vi "Main Abstraction Level 5.vi"() -> ()   [LabVIEW 2019]
doc: "This is one of the levels of abstract design along the timeline leading to the goal of a complete measurement application."
uses:
  messages/MeasureAndLogMessage.lvclass/MeasureAndLogMessage.ctl
  subVIs/Measure and Log Settings.ctl
  subVIs/Simulated Signal Type.ctl
  <extravilib>/ChannelInstances/Stream-str/Read With Abort.vi
  <extravilib>/ChannelInstances/Lossy Stream-a[.](wfm(dbl))/Read With Abort.vi
  <resource>/Channels/Messenger/Read With Abort.vi
  <vilib>/ChannelSupport/Channel Message/Read ID.vi
  <extravilib>/ChannelInstances/Stream-a[.](wfm(dbl))/Read With Abort.vi
  <extravilib>/ChannelInstances/Stream-a[.](wfm(dbl))/Endpoint.vi
  <extravilib>/ChannelInstances/Stream-str/EndpointRead.vi
  <extravilib>/ChannelInstances/Lossy Stream-a[.](wfm(dbl))/EndpointRead.vi
  <extravilib>/ChannelInstances/Stream-a[.](wfm(dbl))/EndpointRead.vi
  <extravilib>/ChannelInstances/Lossy Stream-a[.](wfm(dbl))/Endpoint.vi
  <extravilib>/ChannelInstances/Stream-str/Endpoint.vi
  messages/MeasureAndLogMessage.lvclass
  e:/builds/penguin/labview/branches/2019/dev/dist/vi.lib/ChannelSupport/Channel Message/Channel Message.lvclass
  <extravilib>/ChannelInstances/Tag-path/Instantiate.vi
  <extravilib>/ChannelInstances/Stream-a[.](wfm(dbl))/Instantiate.vi
  <extravilib>/ChannelInstances/Lossy Stream-a[.](wfm(dbl))/Instantiate.vi
  <extravilib>/ChannelInstances/Lossy Stream-a[.](wfm(dbl))/)Channel.vi
  <resource>/ChannelSupport/_ChannelSupport/WaitIfNeeded.vi
  <extravilib>/ChannelInstances/Stream-str/Instantiate.vi
  <extravilib>/ChannelInstances/Stream-str/)Channel.vi
  <extravilib>/ChannelInstances/Tag-bool/Instantiate.vi
  <extravilib>/ChannelInstances/Tag-t'Measure and Log Settings.ctl'/Instantiate.vi
  <resource>/Channels/Messenger/Instantiate.vi
  <resource>/Channels/Messenger/Endpoint.vi
  <extravilib>/ChannelInstances/Tag-t'Measure and Log Settings.ctl'/Endpoint.vi
  <extravilib>/ChannelInstances/Tag-path/Endpoint.vi
  <extravilib>/ChannelInstances/Tag-bool/Endpoint.vi
  <extravilib>/ChannelInstances/Stream-a[.](wfm(dbl))/)Channel.vi
  <resource>/Channels/Messenger/Messenger.lvlib
  <extravilib>/ChannelInstances/Stream-str.lvlib
  <extravilib>/ChannelInstances/Lossy Stream-a[.](wfm(dbl)).lvlib
  <extravilib>/ChannelInstances/Tag-bool.lvlib
  <extravilib>/ChannelInstances/Stream-a[.](wfm(dbl)).lvlib
  <extravilib>/ChannelInstances/Tag-path.lvlib
  <extravilib>/ChannelInstances/Tag-t'Measure and Log Settings.ctl'.lvlib
panel:
  in  "Exit flag":bool
  in  "Record":bool
  in  "Stop":bool
  out "Data":waveform(dbl)[](graph)
  out "Status":string
  in  "Settings":bool
  in  "Start":bool
  in  "Exit":bool
  # "Continuous Measurement Data Logger"
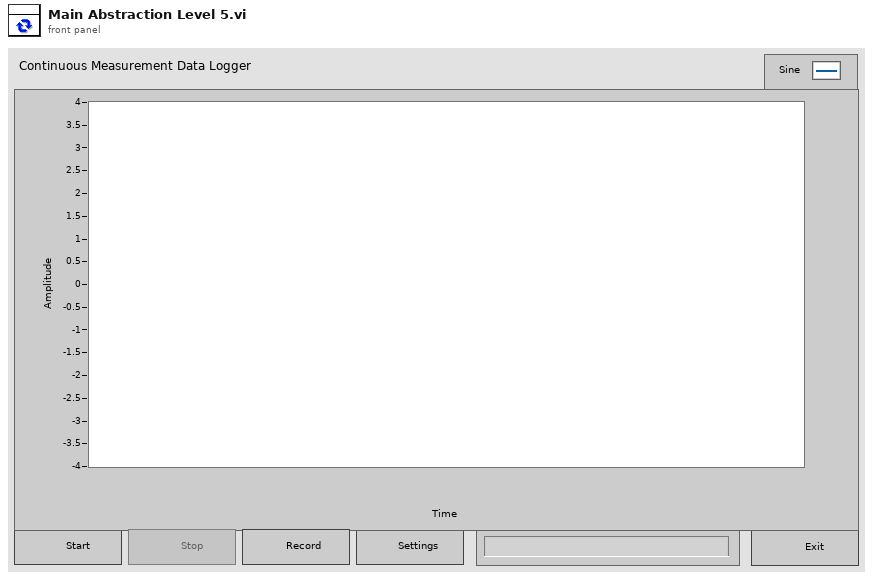
[diagram p1: front panel]
types:
  T1 = typedef "Measure and Log Settings.ctl" = cluster{"sample rate":dbl, "input range":dbl, "logfile path":path, "Simulated Signal":cluster{"signal type":T2, "frequency":dbl, "amplitude":dbl}}
  T2 = typedef "Simulated Signal Type.ctl" = enum16{"Sine Wave", "Square Wave with Noise"}
  T3 = enum8{"Enabled", "Disabled", "Disabled and Grayed Out"}
  T4 = typedef "Messenger.lvlib/))Channel.ctl" = refnum<queue>
  T5 = typedef "Tag-t'Measure and Log Settings.ctl'.lvlib/))Channel.ctl" = refnum<queue>
  T6 = typedef "Tag-path.lvlib/))Channel.ctl" = refnum<queue>
  T7 = typedef "Tag-bool.lvlib/))Channel.ctl" = refnum<queue>
  T8 = typedef "Stream-a[.](wfm(dbl)).lvlib/)Channel.ctl" = refnum<queue>
  T9 = typedef "Stream-str.lvlib/)Channel.ctl" = refnum<queue>
  T10 = typedef "Lossy Stream-a[.](wfm(dbl)).lvlib/)Channel.ctl" = refnum<queue>
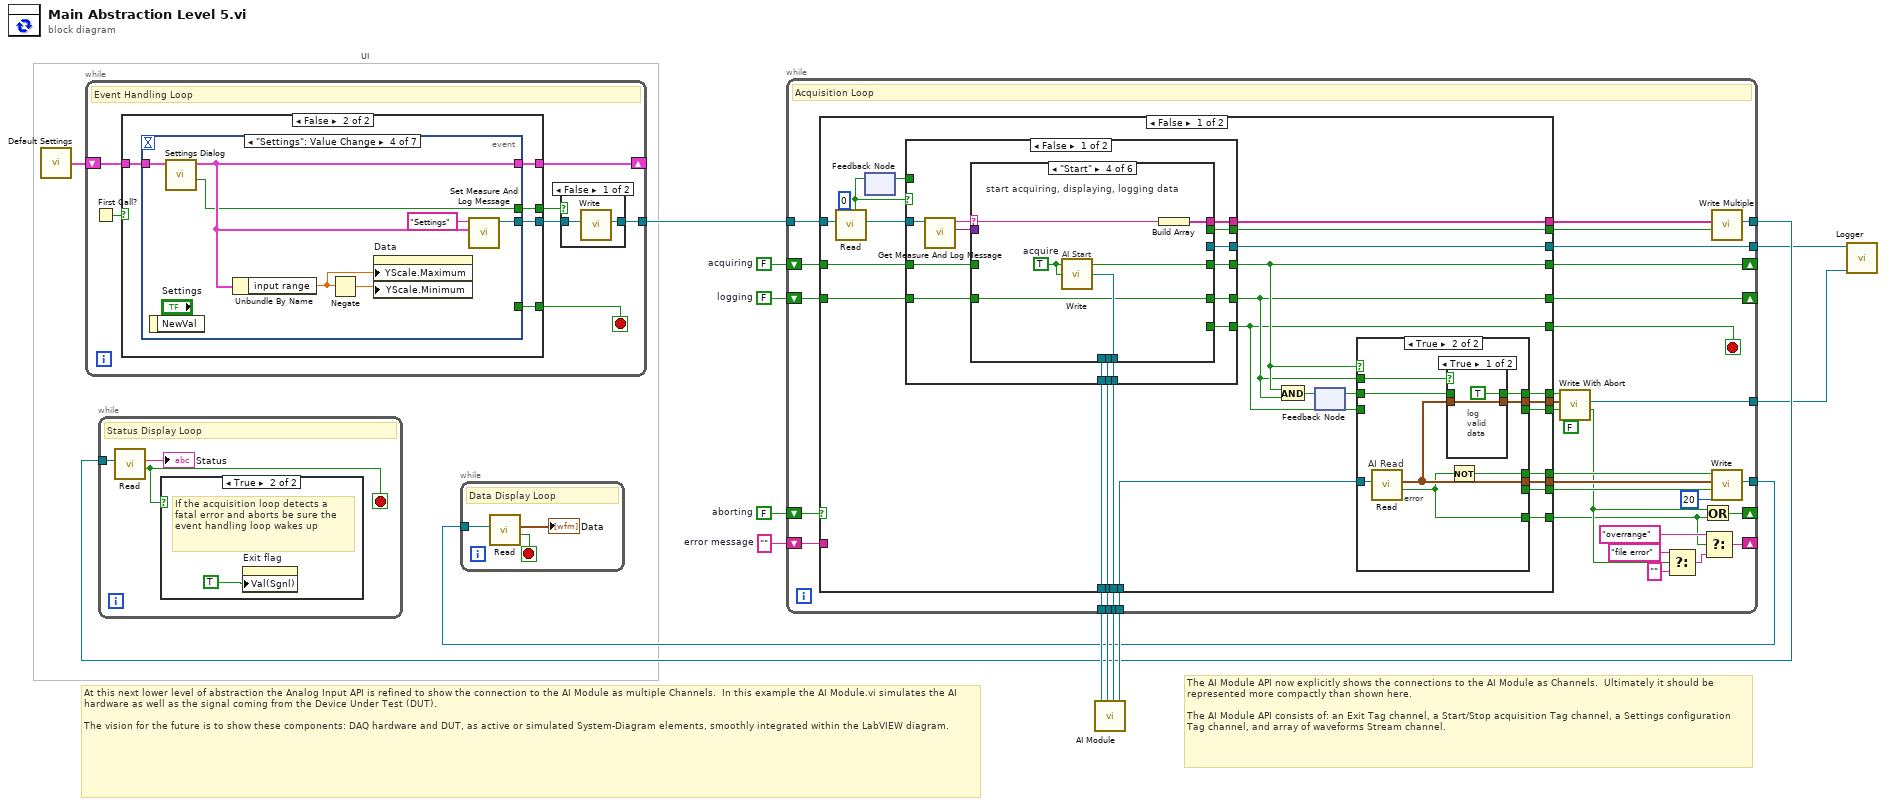
[diagram p0: block diagram]
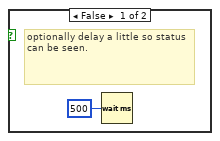
[diagram p2: hidden frame]
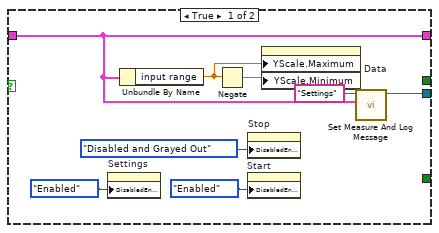
[diagram p3: hidden frame]
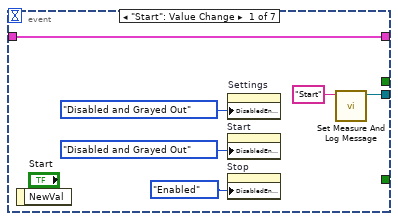
[diagram p4: hidden frame]
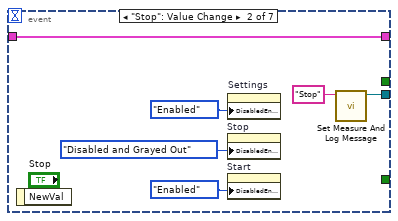
[diagram p5: hidden frame]
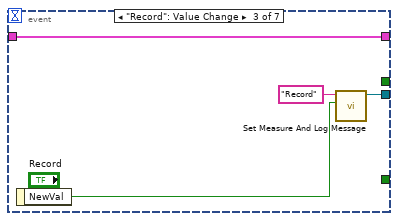
[diagram p6: hidden frame]
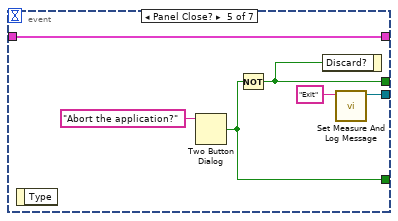
[diagram p7: hidden frame]
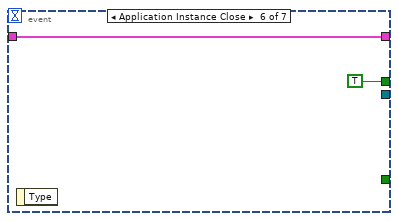
[diagram p8: hidden frame]
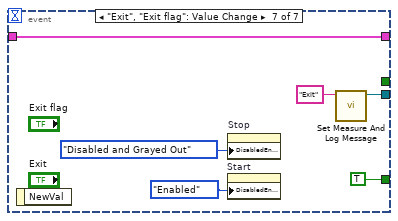
[diagram p9: hidden frame]
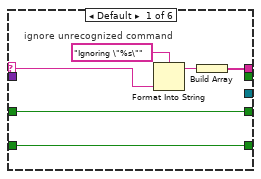
[diagram p11: hidden frame]
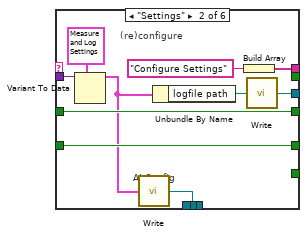
[diagram p12: hidden frame]
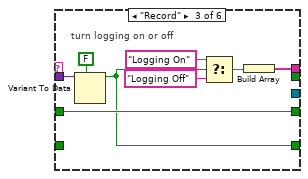
[diagram p13: hidden frame]
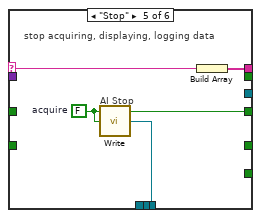
[diagram p14: hidden frame]
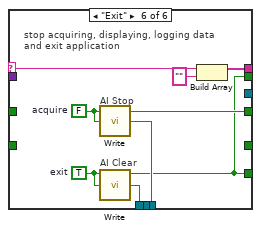
[diagram p15: hidden frame]
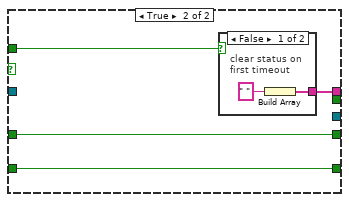
[diagram p16: hidden frame]
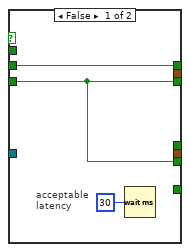
[diagram p18: hidden frame]
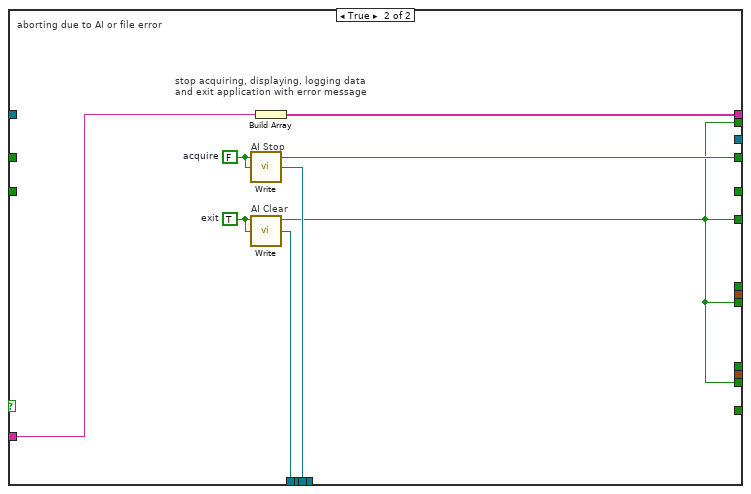
[diagram p20: hidden frame]
diagram:
  w8 = ""  # error message
  w10 = FALSE  # aborting
  w11 = FALSE  # logging
  w12 = FALSE  # acquiring
  # "At this next lower level of abstraction the Analog Input API is refined to show the connection to the AI Module as multiple Channels.  In this example the AI Module.vi simulates the AI hardware as well as the signal coming from the Device Under Test (DUT).\n\nThe vision for the future is to show these components: DAQ hardware and DUT, as active or simulated System-Diagram elements, smoothly integrated within the LabVIEW diagram."
  # "The AI Module API now explicitly shows the connections to the AI Module as Channels.  Ultimately it should be represented more compactly than shown here.\n\nThe AI Module API consists of: an Exit Tag channel, a Start/Stop acquisition Tag channel, a Settings configuration Tag channel, and array of waveforms Stream channel."
  # "UI"
  n1 = call "Default Settings.vi"() -> ("default settings"=w9:T1)
  n2 = while {
    tunnel: [w17] -> w13
    shift-right: [w20] -> _
    shift-left: w9 -> [w19]
    stop <- w21 stop-if-true
    # "Event Handling Loop"
    n3 = First Call?() -> (First Call?: T/F=w18:bool)
    n4 = case shown="False" w18 {
      tunnel: [_ w34] -> w21
      tunnel: [w28 w33] -> w20
      tunnel: w19 -> [w28 w32]
      tunnel: [w24 w31] -> w16
      tunnel: [_ w30] -> w15
      frame True {
        n5 = property on="Settings" class="Bool"("DisabledEnum"=T3."Enabled" ("Disabled")) -> ()  [unwired: 2 in, 2 out]
        n6 = Unbundle By Name(w28) -> ("input range"=w22:dbl)
        n7 = Negate(x=w22) -> (-x=w23:dbl)
        n8 = property on="Stop" class="Bool"("DisabledEnum"=T3."Disabled and Grayed Out" ("Disabled")) -> ()  [unwired: 2 in, 2 out]
        n9 = property on="Start" class="Bool"("DisabledEnum"=T3."Enabled" ("Disabled")) -> ()  [unwired: 2 in, 2 out]
        n10 = property on="Data" class="WFChart (strict)"("YScale.Maximum"=w22, "YScale.Minimum"=w23) -> ()  [unwired: 2 in, 2 out]
        n11 = call "Set Measure And Log Message.vi"("args"=w28, "command"="Settings") -> ("MyMessage"=w24:refnum<class "MeasureAndLogMessage.lvclass">)  [unwired: 9 in]
      }
      frame False {
        n12 = event shown="[3] \"Settings\": Value Change" {
          selector: _ -> [_ _ _ _ _ _ _]
          dyn-events: _ -> [_ _ _ _ _ _ _]
          timeout: _ -> [_ _ _ _ _ _ _]
          tunnel: [_ _ _ _ w59 _ TRUE] -> w34
          tunnel: [w36 w42 w48 w56 w62 w65 w67] -> w33
          tunnel: w32 -> [w36 w42 w48 w57 w62 w65 w67]
          tunnel: [w35 w41 w47 w55 w60 _ w66] -> w31
          tunnel: [_ _ _ w53 w58 TRUE ("cancelled") _] -> w30
          event "Start": Value Change {
            n13 = event-data() -> ()  [unwired: 1 in, 1 out]
            n14 = property on="Settings" class="Bool"("DisabledEnum"=T3."Disabled and Grayed Out" ("Disabled")) -> ()  [unwired: 2 in, 2 out]
            n15 = property on="Start" class="Bool"("DisabledEnum"=T3."Disabled and Grayed Out" ("Disabled")) -> ()  [unwired: 2 in, 2 out]
            n16 = property on="Stop" class="Bool"("DisabledEnum"=T3."Enabled" ("Disabled")) -> ()  [unwired: 2 in, 2 out]
            n17 = call "Set Measure And Log Message.vi"("command"="Start") -> ("MyMessage"=w35:refnum<class "MeasureAndLogMessage.lvclass">)  [unwired: 10 in]
          }
          event "Stop": Value Change {
            n18 = event-data() -> ()  [unwired: 1 in, 1 out]
            n19 = property on="Settings" class="Bool"("DisabledEnum"=T3."Enabled" ("Disabled")) -> ()  [unwired: 2 in, 2 out]
            n20 = property on="Stop" class="Bool"("DisabledEnum"=T3."Disabled and Grayed Out" ("Disabled")) -> ()  [unwired: 2 in, 2 out]
            n21 = property on="Start" class="Bool"("DisabledEnum"=T3."Enabled" ("Disabled")) -> ()  [unwired: 2 in, 2 out]
            n22 = call "Set Measure And Log Message.vi"("command"="Stop") -> ("MyMessage"=w41:refnum<class "MeasureAndLogMessage.lvclass">)  [unwired: 10 in]
          }
          event "Record": Value Change {
            n23 = event-data() -> ("NewVal"=w49:bool)  [unwired: 1 in]
            n24 = call "Set Measure And Log Message.vi"("args"=w49, "command"="Record") -> ("MyMessage"=w47:refnum<class "MeasureAndLogMessage.lvclass">)  [unwired: 9 in]
          }
          event "Settings": Value Change {
            n25 = event-data() -> ()  [unwired: 1 in, 1 out]
            n26 = call "Settings Dialog.vi"("settings in"=w57) -> ("cancelled"=w53:bool, "settings out"=w56:T1)  [unwired: 9 in]
            n27 = Unbundle By Name(w56) -> ("input range"=w51:dbl)
            n28 = Negate(x=w51) -> (-x=w52:dbl)
            n29 = property on="Data" class="WFChart (strict)"("YScale.Maximum"=w51, "YScale.Minimum"=w52) -> ()  [unwired: 2 in, 2 out]
            n30 = call "Set Measure And Log Message.vi"("args"=w56, "command"="Settings") -> ("MyMessage"=w55:refnum<class "MeasureAndLogMessage.lvclass">)  [unwired: 9 in]
          }
          event Panel Close? {
            n31 = event-data() -> ()  [unwired: 1 in, 1 out]
            n32 = Two Button Dialog(message="Abort the application?") -> (T button?=w59:bool)  [unwired: 2 in]
            n33 = Not(x=w59) -> (.not. x?=w58:bool)
            n34 = event-data("Discard?"=w58) -> ()  [unwired: 1 in, 1 out]
            n35 = call "Set Measure And Log Message.vi"("command"="Exit") -> ("MyMessage"=w60:refnum<class "MeasureAndLogMessage.lvclass">)  [unwired: 10 in]
          }
          event Application Instance Close {
            n36 = event-data() -> ()  [unwired: 1 in, 1 out]
          }
          event "Exit", "Exit flag": Value Change {
            n37 = event-data() -> ()  [unwired: 1 in, 1 out]
            n38 = property on="Stop" class="Bool"("DisabledEnum"=T3."Disabled and Grayed Out" ("Disabled")) -> ()  [unwired: 2 in, 2 out]
            n39 = property on="Start" class="Bool"("DisabledEnum"=T3."Enabled" ("Disabled")) -> ()  [unwired: 2 in, 2 out]
            n40 = call "Set Measure And Log Message.vi"("command"="Exit") -> ("MyMessage"=w66:refnum<class "MeasureAndLogMessage.lvclass">)  [unwired: 10 in]
          }
        }
      }
    }
    n41 = case shown="False" w15 {
      tunnel: [w73 _] -> w17
      tunnel: w16 -> [w72 _]
      frame False {
        n42 = call <extravilib>:"Write.vi"("element"=w72) -> ("channel"=w73:T4)  [unwired: 8 in, 2 out]
      }
      frame True {
      }
    }
  }
  n43 = while {
    tunnel: w4 -> [w76]
    stop <- w74 stop-if-true
    # "Status Display Loop"
    n44 = call <extravilib>:"Read.vi"("channel"=w76) -> ("last element?"=w74:bool, "element"=→"Status":string)  [unwired: 6 in, 3 out]
    n45 = case shown="True" w74 {
      frame False {
        # "optionally delay a little so status can be seen."
        n46 = Wait (ms)(milliseconds to wait=u32 500) -> ()  [unwired: 1 out]
      }
      frame True {
        # "If the acquisition loop detects a fatal error and aborts be sure the event handling loop wakes up"
        n47 = property on="Exit flag" class="Bool (strict)"("Val(Sgnl)"=TRUE) -> ()  [unwired: 2 in, 2 out]
      }
    }
  }
  n48 = while {
    tunnel: w3 -> [w79]
    stop <- w81 stop-if-true
    # "Data Display Loop"
    n49 = call <extravilib>:"Read.vi"("channel"=w79) -> ("last element?"=w81:bool, "element"=→"Data":waveform(dbl)[])  [unwired: 5 in, 4 out]
  }
  n50 = while {
    tunnel: w13 -> [w114]
    tunnel: [w102] -> w4
    tunnel: [w99] -> w3
    tunnel: [w95] -> w2
    tunnel: [w110] -> w7
    tunnel: w14 -> [w113]
    shift-right: [w107] -> _
    shift-left: w12 -> [w108]
    shift-right: [w106] -> _
    shift-left: w11 -> [w115]
    tunnel: [w112] -> w1
    tunnel: [w111] -> w6
    tunnel: [w109] -> w5
    shift-right: [w94] -> _
    shift-left: w10 -> [w105]
    shift-right: [w85] -> _
    shift-left: w8 -> [w104]
    stop <- w103 stop-if-true
    # "Acquisition Loop"
    n51 = case shown="False" w105 {
      tunnel: w115 -> [w141 _]
      tunnel: w114 -> [w140 _]
      tunnel: w113 -> [w138 _]
      tunnel: [w134 _] -> w112
      tunnel: [w133 _] -> w111
      tunnel: [w132 w220] -> w110
      tunnel: [w131 w219] -> w109
      tunnel: w108 -> [w130 _]
      tunnel: [w129 w221] -> w107
      tunnel: [w128 _] -> w106
      tunnel: [w125 w216] -> w103
      tunnel: w104 -> [_ w218]
      tunnel: [w123 w216] -> w101
      tunnel: [w124 w217] -> w100
      tunnel: [w121 w216] -> w98
      tunnel: [w122 _] -> w97
      tunnel: [w120 _] -> w96
      tunnel: [w119 _] -> w86
      tunnel: [w118 _] -> w93
      tunnel: [w117 w216] -> w92
      tunnel: [w116 _] -> w91
      frame False {
        n52 = call <extravilib>:"Read.vi"("timeout in ms (-1)"=0, "channel"=w140) -> ("element"=w139:refnum<class "Channel Message.lvclass">, "timed out?"=w136:bool)  [unwired: 7 in, 1 out]
        n53 = feedback #1() -> (w135:bool)  [unwired: 1 in]
        n54 = feedback-in #1(w136) -> ()
        n55 = case shown="False" w136 {
          tunnel: w139 -> [w155 _]
          tunnel: [w151 _] -> w132
          tunnel: [w152 _] -> w125
          tunnel: [w150 w199] -> w129
          tunnel: w130 -> [w149 w199]
          tunnel: [w148 w198] -> w128
          tunnel: w141 -> [w147 w198]
          tunnel: w135 -> [_ w197]
          tunnel: [w146 _] -> w134
          tunnel: [w145 _] -> w133
          tunnel: [w144 _] -> w131
          tunnel: [w143 w196] -> w124
          tunnel: [w142 _] -> w123
          frame False {
            n56 = call "Get Measure And Log Message.vi"("MyMessage"=w155) -> ("args"=w153:variant, "command"=w154:string)  [unwired: 7 in, 2 out]
            n57 = case shown="\"Start\"" w154 {
              selector: w154 -> [w161 _ _ w181 w186 w195]
              tunnel: w153 -> [_ w169 w178 _ _ _]
              tunnel: [_ _ _ w184 w188 w192] -> w151
              tunnel: [_ _ _ _ _ w189] -> w152
              tunnel: [w159 w171 w179 w183 w187 w193] -> w150
              tunnel: w149 -> [w159 w171 w179 _ _ _]
              tunnel: [w158 w170 w174 w182 _ _] -> w148
              tunnel: w147 -> [w158 w170 _ w182 _ _]
              tunnel: [_ w166 _ _ _ _] -> w146
              tunnel: [_ w165 _ _ _ _] -> w145
              tunnel: [_ _ _ _ _ w191] -> w144
              tunnel: [w156 w162 w172 w180 w185 w190] -> w143
              tunnel: [_ _ _ _ _ w189] -> w142
              frame Default {
                # "ignore unrecognized command"
                n58 = Format Into String(format string="Ignoring \"%s\"", w161) -> (resulting string=w157:string)  [unwired: 2 in, 1 out]
                n59 = Build Array(w157) -> (w156:string[])
              }
              frame "Settings" {
                # "AI Config"
                # "(re)configure"
                n60 = Variant To Data(type=T1 {"sample rate"=100.0, "input range"=10.0, "logfile path"=path "/Bohr/Users/jeffk/Documents/LabVIEW Data/Logged Data.tdms", "Simulated Signal"={"signal type"=enum."Sine Wave", "frequency"=1000.0, "amplitude"=5.0}} ("settings out"), Variant=w169) -> (data=w168:T1)  [unwired: 1 in, 1 out]
                n61 = call <extravilib>:"Write.vi"("element"=w168) -> ("channel"=w165:T5)  [unwired: 1 out]
                n62 = Unbundle By Name(w168) -> ("logfile path"=w167:path)
                n63 = Build Array("Configure Settings" ("element")) -> (w162:string[])
                n64 = call <extravilib>:"Write.vi"("element"=w167) -> ("channel"=w166:T6)  [unwired: 1 out]
              }
              frame "Record" {
                # "turn logging on or off"
                n65 = Variant To Data(type=FALSE, Variant=w178) -> (data=w174:bool)  [unwired: 1 in, 1 out]
                n66 = Select(t="Logging On", s=w174, f="Logging Off") -> (s? t:f=w173:string)
                n67 = Build Array(w173) -> (w172:string[])
              }
              frame "Start" {
                w183 = TRUE  # acquire
                # "AI Start"
                # "start acquiring, displaying, logging data"
                n68 = call <extravilib>:"Write.vi"("element"=w183) -> ("channel"=w184:T7)  [unwired: 1 out]
                n69 = Build Array(w181) -> (w180:string[])
              }
              frame "Stop" {
                w187 = FALSE  # acquire
                # "AI Stop"
                # "stop acquiring, displaying, logging data"
                n70 = call <extravilib>:"Write.vi"("element"=w187) -> ("channel"=w188:T7)  [unwired: 1 out]
                n71 = Build Array(w186) -> (w185:string[])
              }
              frame "Exit" {
                w193 = FALSE  # acquire
                w189 = TRUE  # exit
                # "AI Clear"
                # "AI Stop"
                # "stop acquiring, displaying, logging data\nand exit application"
                n72 = call <extravilib>:"Write.vi"("element"=w193) -> ("channel"=w192:T7)  [unwired: 1 out]
                n73 = call <extravilib>:"Write.vi"("element"=w189) -> ("channel"=w191:T7)  [unwired: 1 out]
                n74 = Build Array(w195, "" ("element")) -> (w190:string[])
              }
            }
          }
          frame True {
            n75 = case shown="False" w197 {
              tunnel: [w200 _] -> w196
              frame False {
                # "clear status on\nfirst timeout"
                n76 = Build Array(" " ("string")) -> (w200:string[])
              }
              frame True {
              }
            }
          }
        }
        n77 = And(x=w129, y=w128) -> (x .and. y?=w127:bool)
        n78 = feedback #2() -> (w126:bool)  [unwired: 1 in]
        n79 = feedback-in #2(w127) -> ()
        n80 = case shown="True" w129 {
          tunnel: w138 -> [_ w212]
          tunnel: w128 -> [_ w211]
          tunnel: w126 -> [w204 w210]
          tunnel: w125 -> [w203 _]
          tunnel: [_ w208] -> w122
          tunnel: [w203 _] -> w121
          tunnel: [_ w209] -> w120
          tunnel: [_ w205] -> w119
          tunnel: [w204 w206] -> w118
          tunnel: [w203 _] -> w117
          tunnel: [_ w207] -> w116
          frame False {
            # "acceptable\nlatency"
            n81 = Wait (ms)(milliseconds to wait=u32 30) -> ()  [unwired: 1 out]
          }
          frame True {
            # "error"
            # "AI Read"
            n82 = call <extravilib>:"Read.vi"("channel"=w212) -> ("last element?"=w205:bool, "element"=w209:waveform(dbl)[])  [unwired: 6 in, 3 out]
            n83 = case shown="True" w211 {
              tunnel: w209 -> [w214 _]
              tunnel: w210 -> [_ w215]
              tunnel: [w214 _] -> w207
              tunnel: [TRUE w215] -> w206
              frame True {
                # "log \nvalid\ndata"
              }
              frame False {
              }
            }
            n84 = Not(x=w205) -> (.not. x?=w208:bool)
          }
        }
      }
      frame True {
        w221 = FALSE  # acquire
        w216 = TRUE  # exit
        # "aborting due to AI or file error"
        # "AI Clear"
        # "AI Stop"
        # "stop acquiring, displaying, logging data\nand exit application with error message"
        n85 = call <extravilib>:"Write.vi"("element"=w221) -> ("channel"=w220:T7)  [unwired: 1 out]
        n86 = call <extravilib>:"Write.vi"("element"=w216) -> ("channel"=w219:T7)  [unwired: 1 out]
        n87 = Build Array(w218) -> (w217:string[])
      }
    }
    n88 = call <extravilib>:"Write With Abort.vi"("abort"=FALSE, "last element? (F)"=w92, "element"=w91, "element valid? (T)"=w93) -> ("aborted?"=w89:bool, "channel"=w95:T8)  [unwired: 4 in, 2 out]
    n89 = Select(t="file error", s=w89, f="") -> (s? t:f=w84:string)
    n90 = Or(x=w89, y=w86) -> (x .or. y?=w94:bool)
    n91 = Select(t="overrange", s=w86, f=w84) -> (s? t:f=w85:string)
    n92 = call <extravilib>:"Write Multiple.vi"("last element? (F)"=w101, "elements"=w100) -> ("channel"=w102:T9)  [unwired: 6 in, 3 out]
    n93 = call <extravilib>:"Write.vi"("size (1)"=20, "last element? (F)"=w98, "element"=w96, "element valid? (T)"=w97) -> ("channel"=w99:T10)  [unwired: 5 in, 2 out]
  }
  n94 = call "AI Module.vi"("acquire tag"=w7, "configuration tag"=w6, "exit tag"=w5) -> ("wfm data stream"=w14:T8)  [unwired: 7 in, 1 out]
  n95 = call "Logger.vi"("wfm data stream"=w2, "file path tag"=w1) -> ()  [unwired: 9 in, 1 out]
